vi "Handshake.vi"(8 "error in (no error)":errorcluster, 11 "Connection.LocalQueue":refnum<class "Connection.LocalQueue.lvclass">) -> (0 "error out":errorcluster, 3 "Connection.LocalQueue":refnum<class "Connection.LocalQueue.lvclass">)   [LabVIEW 2013]
uses:
  Connection/Connection.lvclass
  Connection.LocalQueue.lvclass
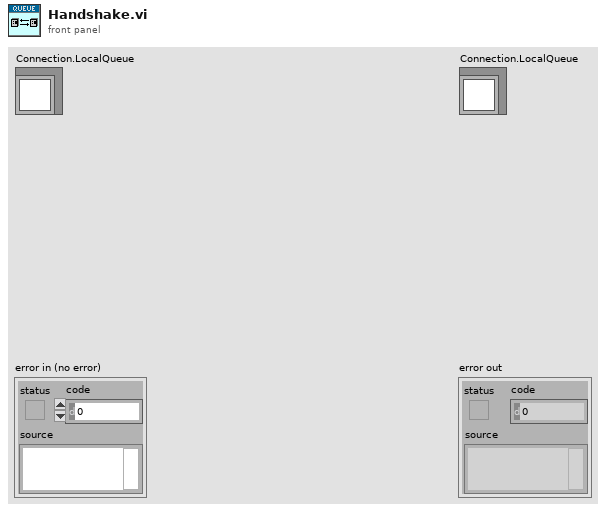
[diagram p1: front panel]
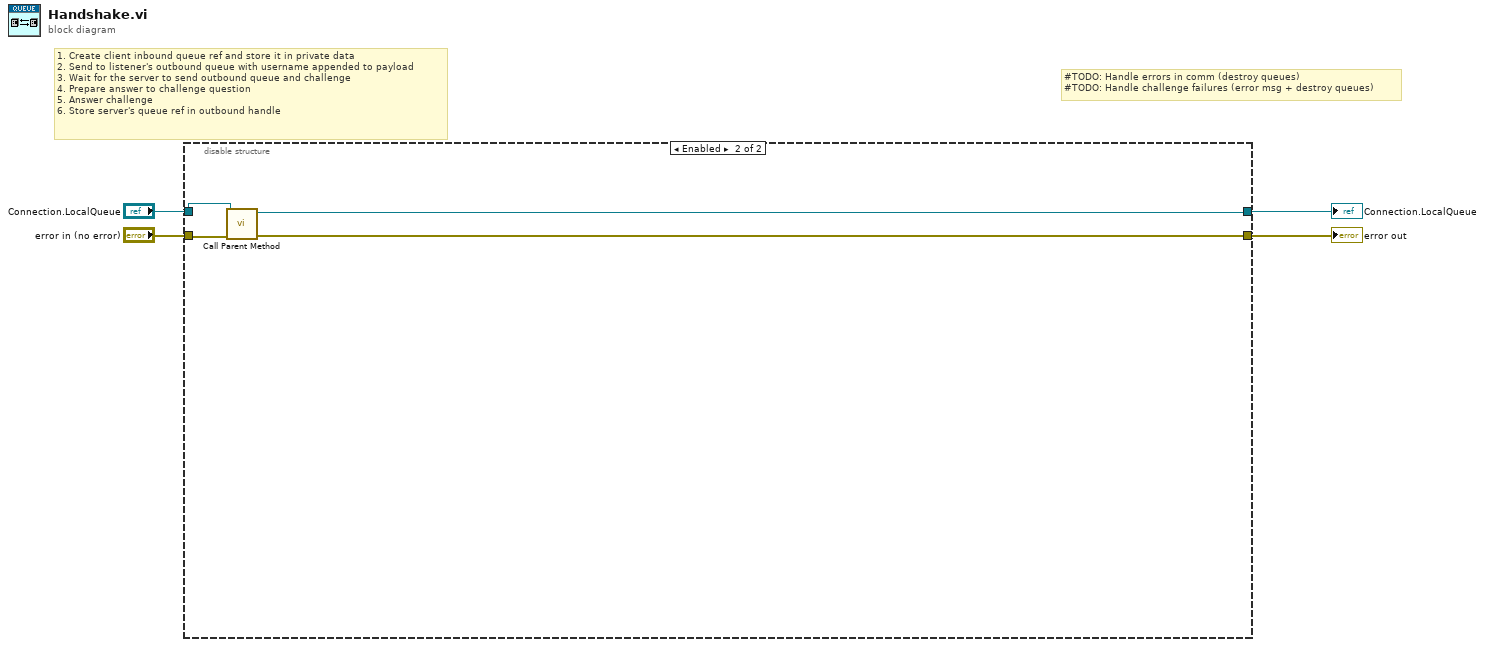
[diagram p0: block diagram]
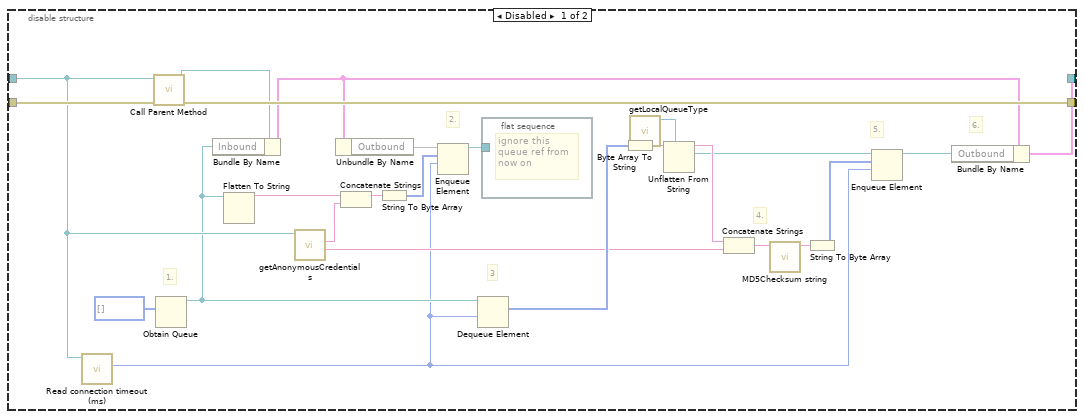
[diagram p2: hidden frame]
diagram:
  # "#TODO: Handle errors in comm (destroy queues)\n#TODO: Handle challenge failures (error msg + destroy queues)"
  # "1. Create client inbound queue ref and store it in private data\n2. Send to listener's outbound queue with username appended to payload\n3. Wait for the server to send outbound queue and challenge\n4. Prepare answer to challenge question\n5. Answer challenge\n6. Store server's queue ref in outbound handle"
  n1 = disable-structure shown="Enabled" {
    disable-tunnel: [w29 w30] -> w4
    disable-tunnel: "error in (no error)" -> [w28 w32]
    disable-tunnel: "Connection.LocalQueue" -> [w18 w33]
    disable-tunnel: [w15 w31] -> w1
    frame Disabled {
      # "6."
      # "5."
      # "4."
      # "3"
      # "2."
      # "1."
      n2 = call "Read connection timeout (ms).vi"("Connection in"=w18) -> ("connection timeout (ms)"=w5:i32)  [unwired: 8 in, 2 out]
      n3 = call-parent "Call Parent Method"("error in (no error)"=w28, "Connection in"=w18) -> ("error out"=w29:errorcluster, "Connection out"=w19:refnum<class "Connection.LocalQueue.lvclass">)  [unwired: 8 in]
      n4 = Obtain Queue(element data type=u8[] [] ("Bytes")) -> (queue out=w17:refnum<queue>)  [unwired: 4 in, 2 out]
      n5 = Bundle By Name(cluster=w19, "Inbound"=w17) -> (w16:cluster{})
      n6 = Flatten To String(anything=w17) -> (data string=w23:string)  [unwired: 3 in, 2 out]
      n7 = call "getAnonymousCredentials.vi"("Connection.LocalQueue"=w18) -> ("Anonymous password"=w11:string, "Anonymous username"=w24:string)  [unwired: 9 in]
      n8 = Unbundle By Name(w16) -> ("Outbound"=w26)
      n9 = Concatenate Strings(w23, w24) -> (w22:string)
      n10 = String To Byte Array(string=w22) -> (unsigned byte array=w25:u8[])
      n11 = Enqueue Element(queue=w26, element=w25, timeout in ms (-1)=w5) -> (queue out=w20:refnum<queue>)  [unwired: 1 in, 2 out]
      n12 = Dequeue Element(queue=w17, timeout in ms (-1)=w5) -> (element=w12:u8[])  [unwired: 1 in, 3 out]
      n13 = flat-sequence {
        tunnel: w20 -> [_]
        frame #0 {
          # "ignore this\nqueue ref from\nnow on"
        }
      }
      n14 = Byte Array To String(unsigned byte array=w12) -> (string=w13:string)
      n15 = call "getLocalQueueType.vi"() -> ("Queue Type"=w14:refnum<queue>)  [unwired: 11 in]
      n16 = Unflatten From String(type=w14, binary string=w13) -> (rest of the binary string=w10:string, value=w9:refnum<queue>)  [unwired: 3 in, 1 out]
      n17 = Concatenate Strings(w10, w11) -> (w21:string)
      n18 = call <vilib>:"MD5Checksum string.vi"("Message String"=w21) -> ("MD5 message-digest"=w7:string)  [unwired: 10 in]
      n19 = String To Byte Array(string=w7) -> (unsigned byte array=w6:u8[])
      n20 = Enqueue Element(queue=w9, element=w6, timeout in ms (-1)=w5) -> (queue out=w8:refnum<queue>)  [unwired: 1 in, 2 out]
      n21 = Bundle By Name(cluster=w16, "Outbound"=w8) -> (w15:cluster{})
    }
    frame Enabled {
      n22 = call-parent "Call Parent Method"("error in (no error)"=w32, "Connection in"=w33) -> ("error out"=w30:errorcluster, "Connection out"=w31:refnum<class "Connection.LocalQueue.lvclass">)  [unwired: 8 in]
    }
  }
  "error out" <- w4
  "Connection.LocalQueue" <- w1
